vi "Set descriptionvi.vi"() -> ()   [LabVIEW 2020]
uses:
  <vilib>/Utility/config.llb/Read Key (String).vi
  <vilib>/Utility/config.llb/NI_LVConfig.lvlib
panel:
  out "section exists?":bool
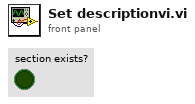
[diagram p1: front panel]
types:
  T1 = typedef "NI_LVConfig.lvlib/Config Data RefNum.ctl" = refnum<k1>
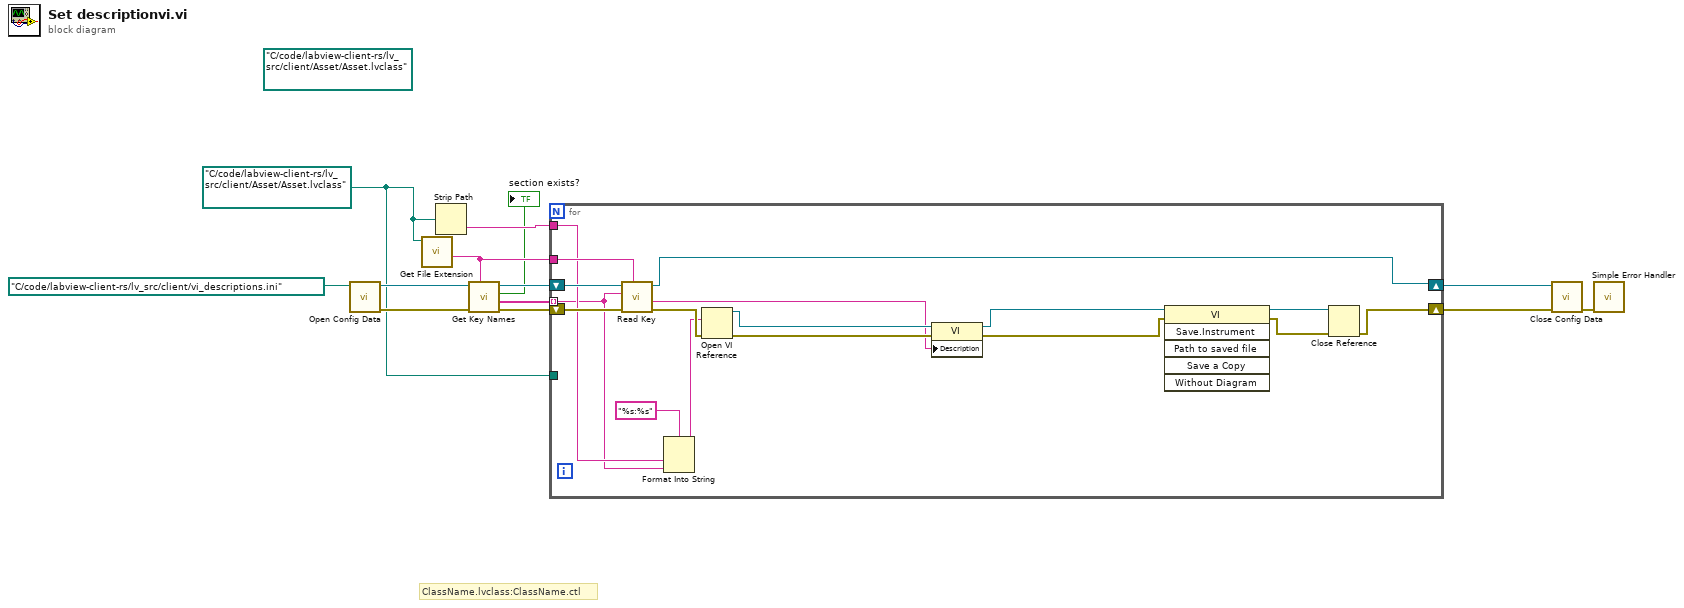
[diagram p0: block diagram]
diagram:
  (unwired) path "C:/code/labview-client-rs/lv_src/client/Asset/Asset.lvclass" ("Path")
  w1 = path "C:/code/labview-client-rs/lv_src/client/Asset/Asset.lvclass" ("Path")
  # "ClassName.lvclass:ClassName.ctl"
  n1 = call <vilib>:"Open Config Data.vi"("configuration file path"=path "C:/code/labview-client-rs/lv_src/client/vi_descriptions.ini") -> ("error out"=w11:errorcluster, "refnum"=w2:T1)  [unwired: 8 in, 1 out]
  n2 = call <vilib>:"Get File Extension.vi"("file"=w1) -> ("filename without extension"=w8:string)  [unwired: 6 in, 4 out]
  n3 = Strip Path(path=w1) -> (name=w6:string)  [unwired: 1 out]
  n4 = call <vilib>:"Get Key Names.vi"("section"=w8, "error in (no error)"=w11, "refnum"=w2) -> ("error out"=w7:errorcluster, "key names"=w10:string[], "section exists?"=→"section exists?":bool, "refnum out"=w9:T1)  [unwired: 5 in]
  n5 = for {
    tunnel: w10 -> [w19] mode=indexing
    tunnel: w8 -> [w28]
    tunnel: w6 -> [w21]
    shift-right: [w26] -> w5
    shift-left: w9 -> [w27]
    shift-right: [w24] -> w4
    shift-left: w7 -> [w25]
    tunnel: w1 -> [_]
    n6 = call-poly <vilib>:"Read Key.vi"("section"=w28, "error in (no error)"=w25, "key"=w19, "refnum"=w27) -> ("error out"=w23:errorcluster, "value"=w14:string, "refnum out"=w26:T1)  [unwired: 4 in, 1 out]
    n7 = Format Into String(format string="%s:%s", w21, w19) -> (resulting string=w20:string)  [unwired: 2 in, 1 out]
    n8 = Open VI Reference(vi path=w20, error in (no error)=w23) -> (vi reference=w16:refnum<vi>, error out=w18:errorcluster)  [unwired: 4 in]
    n9 = property class="VI"(reference=w16, error in=w18, "Description"=w14) -> (reference out=w15:refnum<vi>, error out=w17:errorcluster)
    n10 = invoke class="VI" method="Save.Instrument"(reference=w15, error in=w17) -> (reference out=w29:refnum<vi>, error out=w30:errorcluster)  [unwired: 4 in, 4 out]
    n11 = Close Reference(reference=w29, error in (no error)=w30) -> (error out=w24:errorcluster)
  }
  n12 = call <vilib>:"Close Config Data.vi"("error in (no error)"=w4, "refnum"=w5) -> ("error out"=w13:errorcluster)  [unwired: 8 in, 1 out]
  n13 = call <vilib>:"Simple Error Handler.vi"("error in (no error)"=w13) -> ()  [unwired: 4 in, 5 out]
